vi "Close.vi"(8 "error in (no error)":errorcluster, 11 "NiDaqMx in":refnum<class "NiDaqMx.lvclass">) -> (0 "error out":errorcluster, 3 "NiDaqMx out":refnum<class "NiDaqMx.lvclass">)   [LabVIEW 2018, in "DigitizerPlugins.lvlib" / "NiDaqMx.lvclass"]
uses:
  NiDaqMx.lvclass
  X:/Projects/PMUCal/Modules/Digitizer/DigitizerPlugins/DigitizerBaseClass/DigitizerBase.lvclass
  DigitizerBaseClass/DigitizerBase.lvclass/DigitizerBase.ctl
  NiDaqMx.lvclass/NiDaqMx.ctl
  DigitizerBaseClass/Accessors/Read SyncInfo.vi
  DigitizerBaseClass/Accessors/Read InstRef.vi
  Accessors/Read ExportSignal.vi
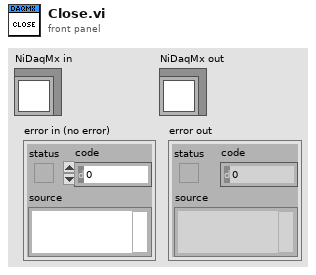
[diagram p1: front panel]
types:
  T1 = typedef "DigitizerPlugins.lvlib/NiDaqMx.lvclass/ExportSignal.ctl" = cluster{"signal":i32, "Destination":string, "Route":string}
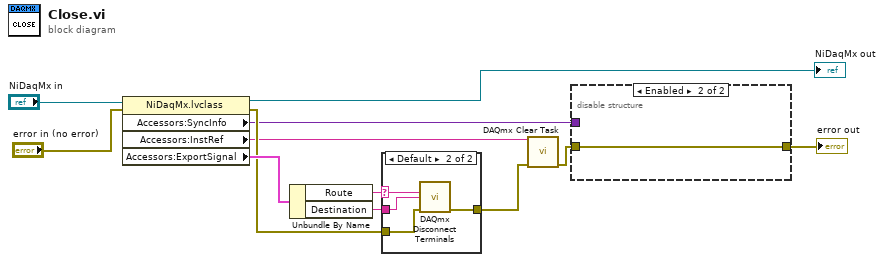
[diagram p0: block diagram]
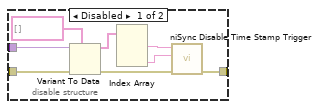
[diagram p2: hidden frame]
diagram:
  n1 = property class="NiDaqMx.lvclass"(reference="NiDaqMx in", error in="error in (no error)") -> (reference out=→"NiDaqMx out":refnum<class "NiDaqMx.lvclass">, error out=w6:errorcluster, "Accessors:SyncInfo"=w2:variant, "Accessors:InstRef"=w4:string, "Accessors:ExportSignal"=w9:T1)
  n2 = Unbundle By Name(w9) -> ("Route"=w7:string, "Destination"=w8:string)
  n3 = case shown="Default" w7 {
    selector: w7 -> [_ w17]
    tunnel: w8 -> [_ w16]
    tunnel: w6 -> [w13 w15]
    tunnel: [w13 w14] -> w5
    frame "", "None", "none" {
    }
    frame Default {
      n4 = call <vilib>:"DAQmx Disconnect Terminals.vi"("source terminal"=w17, "destination terminal"=w16, "error in"=w15) -> ("error out"=w14:errorcluster)  [unwired: 12 in]
    }
  }
  n5 = call <vilib>:"DAQmx Clear Task.vi"("task in"=w4, "error in"=w5) -> ("error out"=w1:errorcluster)  [unwired: 13 in]
  n6 = disable-structure shown="Enabled" {
    disable-tunnel: [w25 w26] -> w3
    disable-tunnel: w2 -> [w24 _]
    disable-tunnel: w1 -> [w23 w26]
    frame Disabled {
      n7 = Variant To Data(error in=w23, type=string[] [], Variant=w24) -> (data=w21:string[], error out=w20:errorcluster)
      n8 = Index Array(array=w21) -> (element #1=w19:string, element #3=w18:string)  [unwired: 3 in, 1 out]
      n9 = call <instrlib>:"niSync Disable Time Stamp Trigger.vi"("error in (no error)"=w20, "terminal"=w18, "instrument handle"=w19) -> ("error out"=w25:errorcluster)  [unwired: 6 in, 1 out]
    }
    frame Enabled {
    }
  }
  "error out" <- w3
